vi "Write Merge in  front.vi"(8 "error in (no error)":errorcluster, 10 "Merge in  front":bool=TRUE, 11 "Combined Measurement in":refnum<class "Combined Measurement.lvclass">) -> (0 "error out":errorcluster, 3 "Combined Measurement out":refnum<class "Combined Measurement.lvclass">)   [LabVIEW 2021, in "Combined Measurement.lvclass"]
uses:
  Combined Measurement.lvclass
  Combined Measurement.lvclass/Combined Measurement.ctl
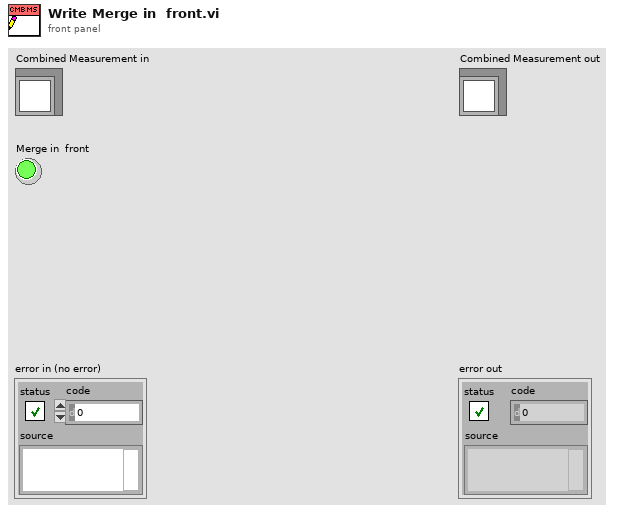
[diagram p1: front panel]
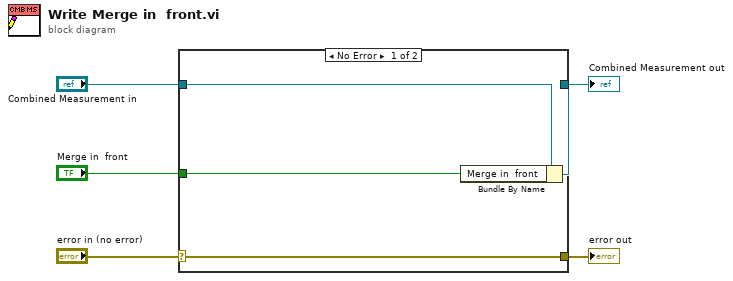
[diagram p0: block diagram]
diagram:
  n1 = case shown="No Error" "error in (no error)" {
    selector: "error in (no error)" -> [w9 w10]
    tunnel: [w9 w10] -> w4
    tunnel: [w7 w11] -> w2
    tunnel: "Combined Measurement in" -> [w8 w11]
    tunnel: "Merge in  front" -> [w6 _]
    frame No Error {
      n2 = Bundle By Name(cluster=w8, "Merge in  front"=w6) -> (w7:refnum<class "Combined Measurement.lvclass">)
    }
    frame Error {
    }
  }
  "error out" <- w4
  "Combined Measurement out" <- w2
